vi "Initialize Discovery.vi"(8 "error in (no error)":errorcluster, 11 "CIFPluginManager in":refnum<class "CIFPluginManager.lvclass">) -> (0 "error out":errorcluster, 3 "CIFPluginManager out":refnum<class "CIFPluginManager.lvclass">)   [LabVIEW 2021, in "CIFPluginManager.lvclass"]
uses:
  CIFPluginManager.lvclass
  CIFPluginManager.lvclass/CIFPluginManager.ctl
  typedef/Plugin Metadata.ctl
  CIFCore/Common/Typedef/Version.ctl
  CIFCore/Common/CIFCoreCommon.lvlib
  typedef/Discovered Plugin.ctl
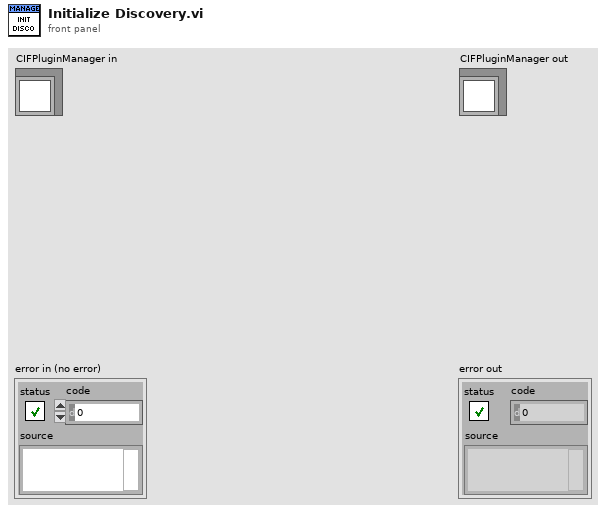
[diagram p1: front panel]
types:
  T1 = typedef "CIFPluginManager.lvclass/Discovered Plugin.ctl" = cluster{"Filename":string, "Plugin Type":string, "Qualified name":string, "Version":T2, "Plugin Metadata":T3}
  T2 = typedef "CIFCoreCommon.lvlib/Version.ctl" = cluster{"Major":i32, "Minor":i32, "Fix":i32, "Build":i32}
  T3 = typedef "CIFPluginManager.lvclass/Plugin Metadata.ctl" = cluster{"Description":string, "History":string, "Author":string}
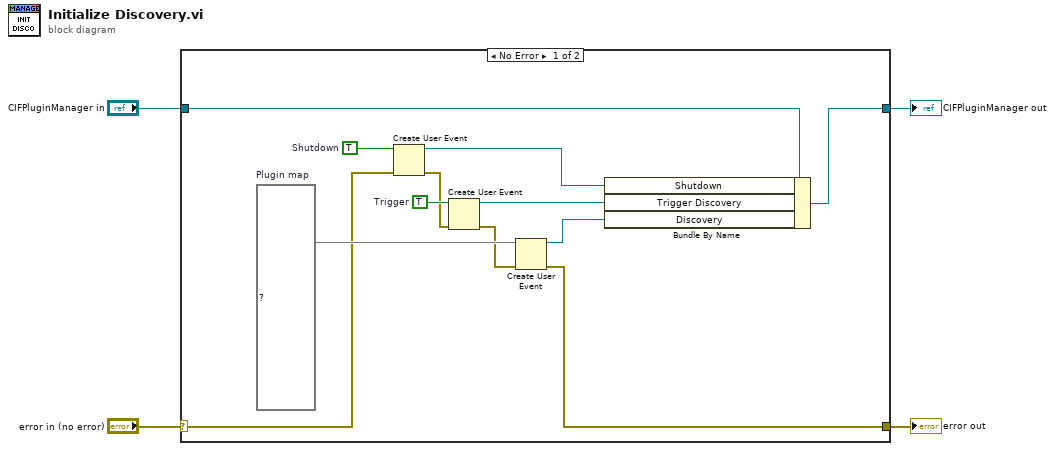
[diagram p0: block diagram]
diagram:
  n1 = case shown="No Error" "error in (no error)" {
    selector: "error in (no error)" -> [w8 w18]
    tunnel: [w9 w18] -> w3
    tunnel: [w15 w17] -> w1
    tunnel: "CIFPluginManager in" -> [w16 w17]
    frame No Error {
      w6 = TRUE  # Shutdown
      w12 = map{string, T1[]} {}  # Plugin map
      w14 = TRUE  # Trigger
      n2 = Create User Event(user event datatype=w6, error in=w8) -> (user event=w5:refnum<user-event>, error out=w7:errorcluster)
      n3 = Create User Event(user event datatype=w14, error in=w7) -> (user event=w13:refnum<user-event>, error out=w10:errorcluster)
      n4 = Create User Event(user event datatype=w12, error in=w10) -> (user event=w11:refnum<user-event>, error out=w9:errorcluster)
      n5 = Bundle By Name(cluster=w16, "Shutdown"=w5, "Trigger Discovery"=w13, "Discovery"=w11) -> (w15:refnum<class "CIFPluginManager.lvclass">)
    }
    frame Error {
    }
  }
  "error out" <- w3
  "CIFPluginManager out" <- w1
